vi "英维克通讯.vi"() -> ()   [LabVIEW 2016, in "环境动力监测库.lvlib" / "空调库.lvlib"]
uses:
  <vilib>/Plasmionique/MB Master/MB_Master/MB_Master.lvclass
  <vilib>/Plasmionique/MB Master/MB Master.lvlib
  <vilib>/Utility/config.llb/NI_LVConfig.lvlib
panel:
  out "遥控开关机状态":bool
  out "系统参数":T1
  out "告警状态":T2
  out "传感器状态":T3
  out "运行状态":T4
  out "遥控参数":u16[](array[numeric])
  out "系统参数":u16[](array[numeric])
  out "告警状态":u16[](array[numeric])
  out "传感器状态":u16[](array[numeric])
  out "运行状态":u16[](array[numeric])
  in  "读取参数":bool
  in  "读取数据":bool
  in  "释放串口":bool
  in  "打开串口":bool
  out "队列中元素数量":i32
  out "元素":cluster{"命令":string}[](array[cluster])
  out "待处理插入数量":i32
  out "读取公式":u16[](array[numeric])
  out "读取参数":u16[](array[numeric])
  out "数据存储":u16[](array[numeric])
  out "通讯状态":bool
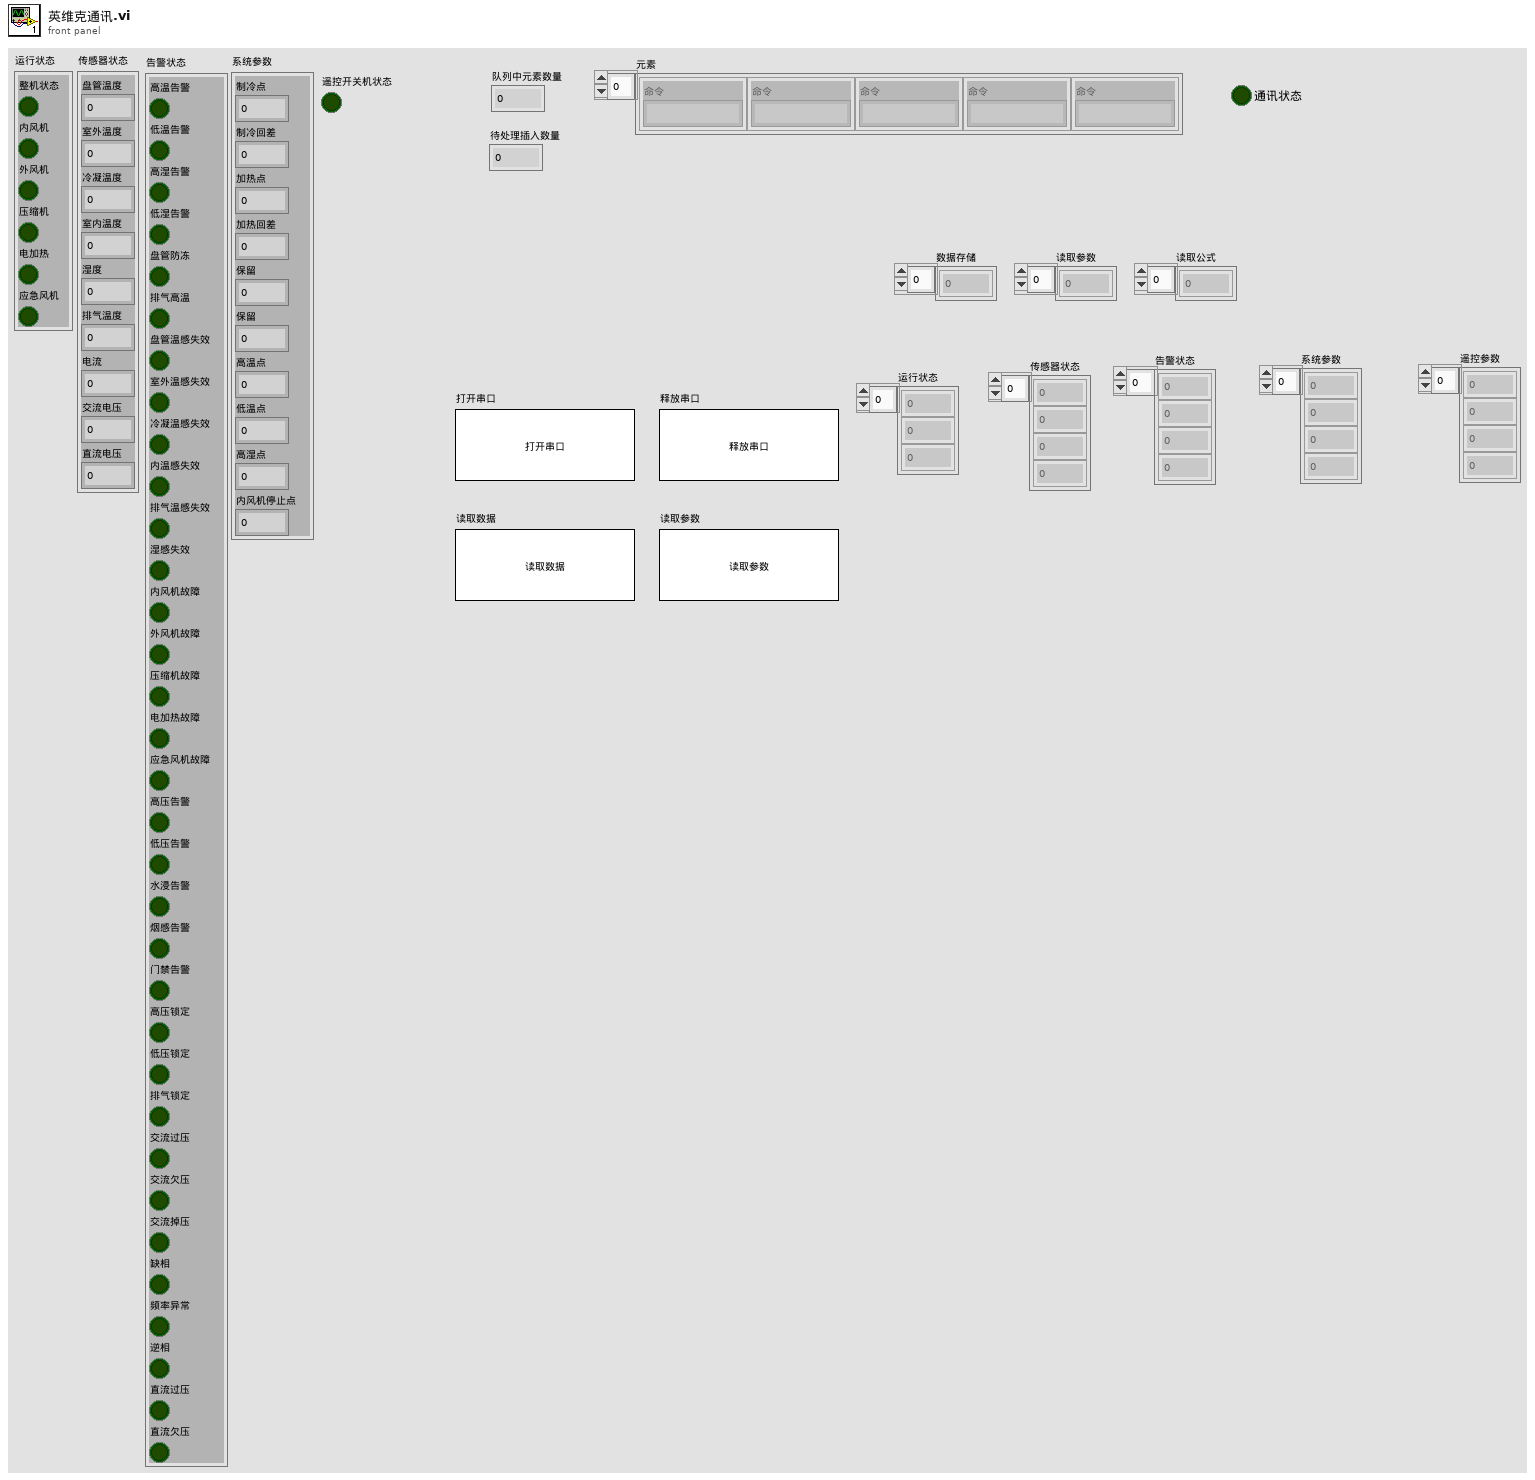
[diagram p1: front panel]
types:
  T1 = cluster{"制冷点":u16, "制冷回差":u16, "加热点":u16, "加热回差":u16, "保留":u16, "保留":u16, "高温点":u16, "低温点":u16, "高湿点":u16, "内风机停止点":u16}
  T2 = cluster{"高温告警":bool, "低温告警":bool, "高湿告警":bool, "低湿告警":bool, "盘管防冻":bool, "排气高温":bool, "盘管温感失效":bool, "室外温感失效":bool, "冷凝温感失效":bool, "内温感失效":bool, "排气温感失效":bool, "湿感失效":bool, "内风机故障":bool, "外风机故障":bool, "压缩机故障":bool, "电加热故障":bool, "应急风机故障":bool, "高压告警":bool, "低压告警":bool, "水浸告警":bool, "烟感告警":bool, "门禁告警":bool, "高压锁定":bool, "低压锁定":bool, "排气锁定":bool, "交流过压":bool, "交流欠压":bool, "交流掉压":bool, "缺相":bool, "频率异常":bool, "逆相":bool, "直流过压":bool, "直流欠压":bool}
  T3 = cluster{"盘管温度":u16, "室外温度":u16, "冷凝温度":u16, "室内温度":u16, "湿度":u16, "排气温度":u16, "电流":u16, "交流电压":u16, "直流电压":u16}
  T4 = cluster{"整机状态":bool, "内风机":bool, "外风机":bool, "压缩机":bool, "电加热":bool, "应急风机":bool}
  T5 = typedef "NI_LVConfig.lvlib/Config Data RefNum.ctl" = refnum<k1>
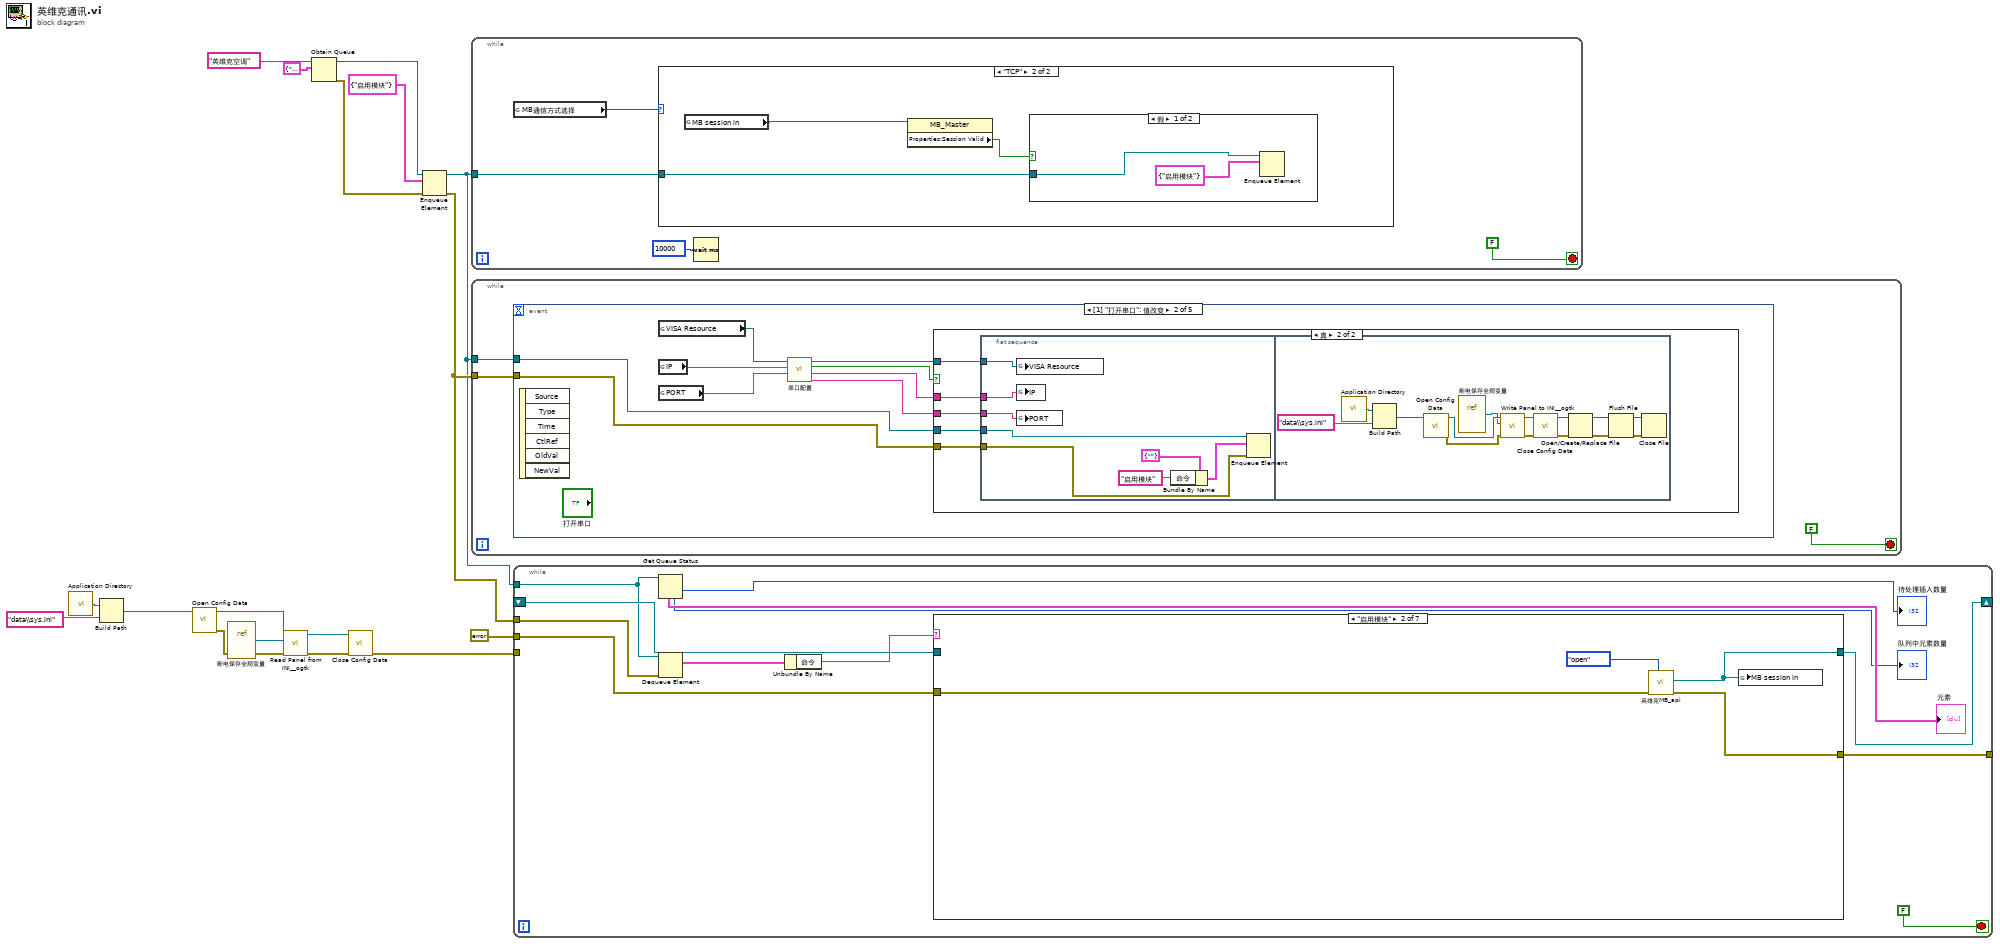
[diagram p0: block diagram]
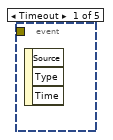
[diagram p4: hidden frame]
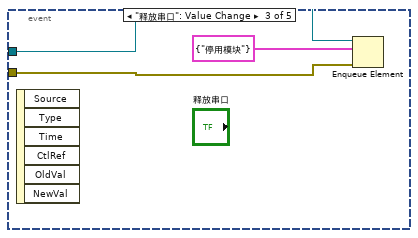
[diagram p6: hidden frame]
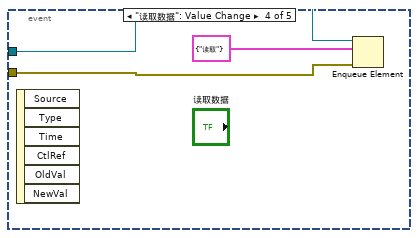
[diagram p7: hidden frame]
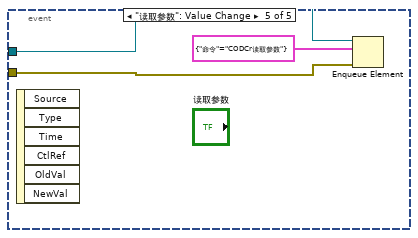
[diagram p8: hidden frame]
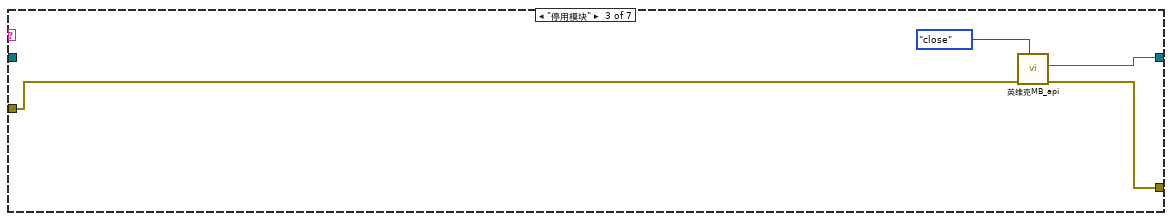
[diagram p10: hidden frame]
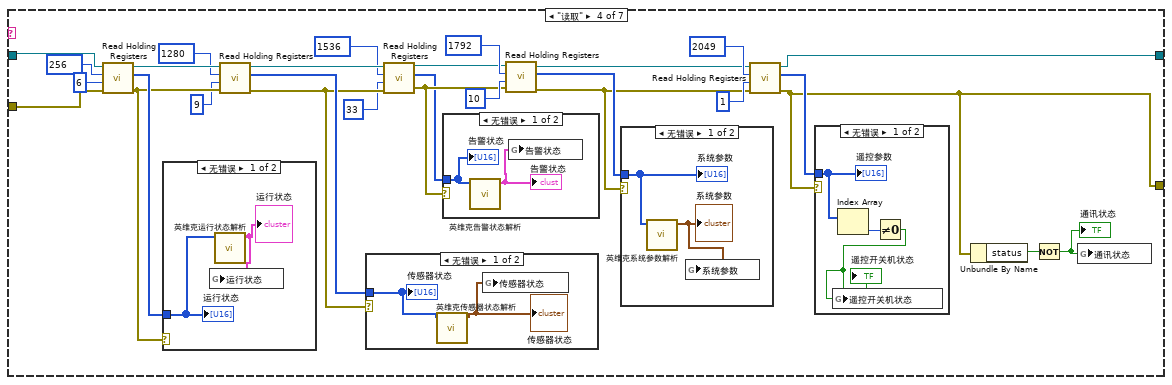
[diagram p11: hidden frame]
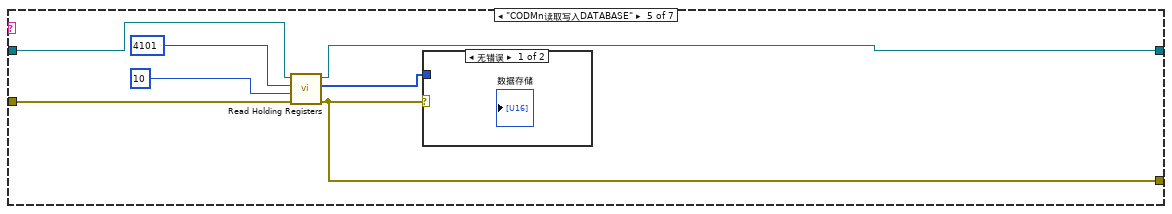
[diagram p17: hidden frame]
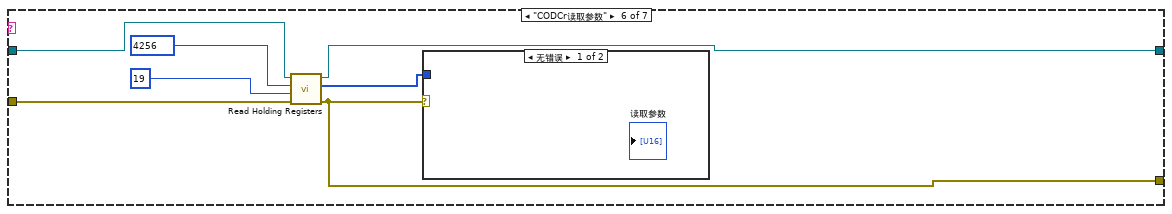
[diagram p19: hidden frame]
diagram:
  n1 = call <vilib>:"Application Directory.vi"() -> ("Application Directory"=w2:path)
  n2 = Build Path(base path=w2, name or relative path="data\\sys.ini" ("名称或相对路径")) -> (appended path=w3:path)
  n3 = call <vilib>:"Open Config Data.vi"("configuration file path"=w3) -> ("error out"=w8:errorcluster, "refnum"=w11:T5)  [unwired: 8 in, 1 out]
  n4 = vi-ref "断电保存全局变量.vi"() -> (w10:refnum<vi>)
  n5 = call <userlib>:"Read Panel from INI__ogtk.vi"("error in (no error)"=w8, "VI ref"=w10, "refnum"=w11) -> ("error out"=w7:errorcluster, "refnum out"=w9:T5)  [unwired: 7 in]
  n6 = Obtain Queue(name (unnamed)="英维克空调" ("名称（未命名）"), element data type=cluster{"命令":string} {"命令"="启用模块"} ("元素")) -> (queue out=w14:refnum<queue>, error out=w13:errorcluster)  [unwired: 3 in, 1 out]
  n7 = call <vilib>:"Close Config Data.vi"("error in (no error)"=w7, "refnum"=w9) -> ("error out"=w4:errorcluster)  [unwired: 8 in, 1 out]
  n8 = Enqueue Element(queue=w14, element=cluster{"命令":string} {"命令"="启用模块"} ("元素"), error in (no error)=w13) -> (queue out=w5:refnum<queue>, error out=w6:errorcluster)  [unwired: 1 in, 1 out]
  n9 = while {
    tunnel: w5 -> [w21]
    stop <- FALSE stop-if-true
    n10 = global read "断电保存全局变量.vi" "MB通信方式选择"() -> (w19:enum16{"串口", "TCP"})
    n11 = case shown="\"TCP\"" w19 {
      tunnel: w21 -> [_ w23]
      frame "串口", Default {
      }
      frame "TCP" {
        n12 = global read "断电保存全局变量.vi" "MB session in"() -> (w22:refnum<class "MB_Master.lvclass">)
        n13 = property class="MB_Master"(reference=w22) -> ("Properties:Session Valid"=w24:bool)  [unwired: 1 in, 2 out]
        n14 = case shown="假" w24 {
          tunnel: w23 -> [w26 _]
          frame False {
            n15 = Enqueue Element(queue=w26, element=cluster{"命令":string} {"命令"="启用模块"} ("元素")) -> ()  [unwired: 2 in, 3 out]
          }
          frame True {
          }
        }
      }
    }
    n16 = Wait (ms)(milliseconds to wait=u32 10000 ("等待时间（毫秒）")) -> ()  [unwired: 1 out]
  }
  n17 = while {
    tunnel: w5 -> [w28]
    tunnel: w6 -> [w27]
    stop <- FALSE stop-if-true
    n18 = event shown="[1] \"打开串口\": 值改变" {
      selector: _ -> [_ _ _ _ _]
      dyn-events: _ -> [_ _ _ _ _]
      timeout: _ -> [_ _ _ _ _]
      tunnel: w28 -> [_ w38 w68 w70 w73]
      tunnel: w27 -> [_ w37 w67 w69 w72]
      event Timeout {
        n19 = event-data() -> ()  [unwired: 1 in, 3 out]
      }
      event "打开串口": Value Change {
        n20 = event-data() -> ()  [unwired: 1 in, 6 out]
        n21 = global read "断电保存全局变量.vi" "VISA Resource"() -> (w36:refnum<visa-resource-name>)
        n22 = global read "断电保存全局变量.vi" "IP"() -> (w31:string)
        n23 = global read "断电保存全局变量.vi" "PORT"() -> (w30:string)
        n24 = call "串口配置.vi"("PORT"=w30, "IP"=w31, "请选择串口:"=w36) -> ("PORT 2"=w32:string, "IP 2"=w33:string, "确认 2"=w34:bool, "VISA资源名称 2"=w35:refnum<visa-resource-name>)  [unwired: 5 in]
        n25 = case shown="真" w34 {
          tunnel: w35 -> [_ w41]
          tunnel: w38 -> [_ w43]
          tunnel: w37 -> [_ w42]
          tunnel: w33 -> [_ w40]
          tunnel: w32 -> [_ w39]
          frame False {
          }
          frame True {
            n26 = flat-sequence {
              tunnel: w43 -> [w48]
              tunnel: w42 -> [w47]
              tunnel: w41 -> [w46]
              tunnel: w40 -> [w45]
              tunnel: w39 -> [w44]
              frame #0 {
                n27 = global write "断电保存全局变量.vi" "VISA Resource"(w46) -> ()
                n28 = global write "断电保存全局变量.vi" "IP"(w45) -> ()
                n29 = global write "断电保存全局变量.vi" "PORT"(w44) -> ()
                n30 = Bundle By Name(cluster=cluster{"命令":string} {"命令"=""} ("元素"), "命令"="启用模块" ("名称（未命名）")) -> (w49:cluster{"命令":string})
                n31 = Enqueue Element(queue=w48, element=w49, error in (no error)=w47) -> ()  [unwired: 1 in, 3 out]
              }
              frame #1 {
                n32 = call <vilib>:"Application Directory.vi"() -> ("Application Directory"=w64:path)
                n33 = Build Path(base path=w64, name or relative path="data\\sys.ini" ("名称或相对路径")) -> (appended path=w63:path)
                n34 = call <vilib>:"Open Config Data.vi"("configuration file path"=w63) -> ("error out"=w59:errorcluster, "refnum"=w62:T5)  [unwired: 8 in, 1 out]
                n35 = vi-ref "断电保存全局变量.vi"() -> (w61:refnum<vi>)
                n36 = call <userlib>:"Write Panel to INI__ogtk.vi"("error in (no error)"=w59, "VI ref"=w61, "refnum"=w62) -> ("error out"=w58:errorcluster, "refnum out"=w60:T5)  [unwired: 7 in]
                n37 = call <vilib>:"Close Config Data.vi"("error in (no error)"=w58, "refnum"=w60) -> ("error out"=w53:errorcluster, "file path"=w52:path)  [unwired: 8 in]
                n38 = Open/Create/Replace File(file path (use dialog)=w52, error in=w53) -> (refnum out=w56:refnum<file>, error out=w57:errorcluster)  [unwired: 4 in, 1 out]
                n39 = Flush File(refnum=w56, error in=w57) -> (refnum out=w55:refnum<file>, error out=w54:errorcluster)
                n40 = Close File(refnum=w55, error in=w54) -> ()  [unwired: 2 out]
              }
            }
          }
        }
      }
      event "释放串口": Value Change {
        n41 = event-data() -> ()  [unwired: 1 in, 6 out]
        n42 = Enqueue Element(queue=w68, element=cluster{"命令":string} {"命令"="停用模块"} ("元素"), error in (no error)=w67) -> ()  [unwired: 1 in, 3 out]
      }
      event "读取数据": Value Change {
        n43 = event-data() -> ()  [unwired: 1 in, 6 out]
        n44 = Enqueue Element(queue=w70, element=cluster{"命令":string} {"命令"="读取"} ("元素"), error in (no error)=w69) -> ()  [unwired: 1 in, 3 out]
      }
      event "读取参数": Value Change {
        n45 = event-data() -> ()  [unwired: 1 in, 6 out]
        n46 = Enqueue Element(queue=w73, element=cluster{"命令":string} {"命令"="CODCr读取参数"} ("元素"), error in (no error)=w72) -> ()  [unwired: 1 in, 3 out]
      }
    }
  }
  n47 = while {
    tunnel: w5 -> [w78]
    tunnel: w6 -> [w85]
    tunnel: [w79] -> _
    shift-right: [w82] -> _
    shift-left: _ -> [w81]
    tunnel: errorcluster {"status"=FALSE, "code"=0, "source"=""} ("error out") -> [w80]
    tunnel: w4 -> [_]
    stop <- FALSE stop-if-true
    n48 = Get Queue Status(queue=w78) -> (# pending insert=→"待处理插入数量":i32, # elements in queue=→"队列中元素数量":i32, elements=→"元素":cluster{"命令":string}[])  [unwired: 2 in, 5 out]
    n49 = Dequeue Element(queue=w78, error in (no error)=w85) -> (element=w84:cluster{"命令":string})  [unwired: 1 in, 3 out]
    n50 = Unbundle By Name(w84) -> ("命令"=w83:string)
    n51 = case shown="\"启用模块\"" w83 {
      tunnel: [w88 w89 w93 w98 w139 w147 w154] -> w82
      tunnel: [w87 w92 w94 w97 w137 w146 w153] -> w79
      tunnel: w81 -> [w88 _ _ w125 w143 w150 w157]
      tunnel: w80 -> [w87 w90 w95 w124 w140 w149 w156]
      frame Default {
      }
      frame "启用模块" {
        n52 = call "英维克MB_api.vi"("STEP"=enum16{"open", "read", "write", "close"}."open", "Error in"=w90) -> ("error out"=w92:errorcluster, "MB session out"=w89:refnum<class "MB_Master.lvclass">)  [unwired: 7 in, 1 out]
        n53 = global write "断电保存全局变量.vi" "MB session in"(w89) -> ()
      }
      frame "停用模块" {
        n54 = call "英维克MB_api.vi"("STEP"=enum16{"open", "read", "write", "close"}."close", "Error in"=w95) -> ("error out"=w94:errorcluster, "MB session out"=w93:refnum<class "MB_Master.lvclass">)  [unwired: 7 in, 1 out]
      }
      frame "读取" {
        n55 = call <vilib>:"Read Holding Registers.vi"("error in (no error)"=w124, "quantity"=u16 6 ("number of holding registers"), "starting address"=u16 256, "MB session in"=w125) -> ("error out"=w121:errorcluster, "Registers"=w123:u16[], "MB session out"=w122:refnum<class "MB_Master.lvclass">)  [unwired: 5 in]
        n56 = case shown="无错误" w121 {
          tunnel: w123 -> [w136 _]
          frame No Error {
            n57 = call "英维克运行状态解析.vi"("运行状态输入"=w136) -> ("运行状态"=w135:T4)  [unwired: 10 in]
            "运行状态" <- w135
            n58 = global write "内部交互全局变量.vi" "运行状态"(w135) -> ()
            "运行状态" <- w136
          }
          frame Error {
          }
        }
        n59 = call <vilib>:"Read Holding Registers.vi"("error in (no error)"=w121, "quantity"=u16 9 ("number of holding registers"), "starting address"=u16 1280, "MB session in"=w122) -> ("error out"=w112:errorcluster, "Registers"=w120:u16[], "MB session out"=w113:refnum<class "MB_Master.lvclass">)  [unwired: 5 in]
        n60 = case shown="无错误" w112 {
          tunnel: w120 -> [w134 _]
          frame No Error {
            n61 = call "英维克传感器状态解析.vi"("传感器状态输入"=w134) -> ("传感器状态输出"=w133:T3)  [unwired: 10 in]
            "传感器状态" <- w133
            n62 = global write "内部交互全局变量.vi" "传感器状态"(w133) -> ()
            "传感器状态" <- w134
          }
          frame Error {
          }
        }
        n63 = call <vilib>:"Read Holding Registers.vi"("error in (no error)"=w112, "quantity"=u16 33 ("number of holding registers"), "starting address"=u16 1536, "MB session in"=w113) -> ("error out"=w106:errorcluster, "Registers"=w105:u16[], "MB session out"=w107:refnum<class "MB_Master.lvclass">)  [unwired: 5 in]
        n64 = case shown="无错误" w106 {
          tunnel: w105 -> [w132 _]
          frame No Error {
            n65 = call "英维克告警状态解析.vi"("告警状态输入"=w132) -> ("告警状态"=w131:T2)  [unwired: 10 in]
            "告警状态" <- w131
            n66 = global write "内部交互全局变量.vi" "告警状态"(w131) -> ()
            "告警状态" <- w132
          }
          frame Error {
          }
        }
        n67 = call <vilib>:"Read Holding Registers.vi"("error in (no error)"=w106, "quantity"=u16 10 ("number of holding registers"), "starting address"=u16 1792, "MB session in"=w107) -> ("error out"=w101:errorcluster, "Registers"=w104:u16[], "MB session out"=w100:refnum<class "MB_Master.lvclass">)  [unwired: 5 in]
        n68 = case shown="无错误" w101 {
          tunnel: w104 -> [w130 _]
          frame No Error {
            n69 = call "英维克系统参数解析.vi"("系统参数输入"=w130) -> ("系统参数"=w129:T1)  [unwired: 10 in]
            "系统参数" <- w129
            n70 = global write "内部交互全局变量.vi" "系统参数"(w129) -> ()
            "系统参数" <- w130
          }
          frame Error {
          }
        }
        n71 = call <vilib>:"Read Holding Registers.vi"("error in (no error)"=w101, "quantity"=u16 1 ("number of holding registers"), "starting address"=u16 2049, "MB session in"=w100) -> ("error out"=w97:errorcluster, "Registers"=w99:u16[], "MB session out"=w98:refnum<class "MB_Master.lvclass">)  [unwired: 5 in]
        n72 = case shown="无错误" w97 {
          tunnel: w99 -> [w128 _]
          frame No Error {
            n73 = Index Array(array=w128) -> (element=w127:u16)  [unwired: 1 in]
            n74 = Not Equal To 0?(x=w127) -> (x != 0?=w126:bool)
            "遥控开关机状态" <- w126
            n75 = global write "内部交互全局变量.vi" "遥控开关机状态"(w126) -> ()
            "遥控参数" <- w128
          }
          frame Error {
          }
        }
        n76 = Unbundle By Name(w97) -> ("status"=w114:bool)
        n77 = Not(x=w114) -> (.not. x?=w115:bool)
        "通讯状态" <- w115
        n78 = global write "断电保存全局变量.vi" "通讯状态"(w115) -> ()
      }
      frame "CODMn读取写入DATABASE" {
        n79 = call <vilib>:"Read Holding Registers.vi"("error in (no error)"=w140, "quantity"=u16 10 ("number of holding registers"), "starting address"=u16 4101, "MB session in"=w143) -> ("error out"=w137:errorcluster, "Registers"=w138:u16[], "MB session out"=w139:refnum<class "MB_Master.lvclass">)  [unwired: 5 in]
        n80 = case shown="无错误" w137 {
          tunnel: w138 -> [_ _]
          frame No Error {
          }
          frame Error {
          }
        }
      }
      frame "CODCr读取参数" {
        n81 = call <vilib>:"Read Holding Registers.vi"("error in (no error)"=w149, "quantity"=u16 19 ("number of holding registers"), "starting address"=u16 4256, "MB session in"=w150) -> ("error out"=w146:errorcluster, "Registers"=w148:u16[], "MB session out"=w147:refnum<class "MB_Master.lvclass">)  [unwired: 5 in]
        n82 = case shown="无错误" w146 {
          tunnel: w148 -> [_ _]
          frame No Error {
          }
          frame Error {
          }
        }
      }
      frame "CODMn读取公式" {
        n83 = call <vilib>:"Read Holding Registers.vi"("error in (no error)"=w156, "quantity"=u16 94 ("number of holding registers"), "starting address"=u16 4616, "MB session in"=w157) -> ("error out"=w153:errorcluster, "Registers"=w155:u16[], "MB session out"=w154:refnum<class "MB_Master.lvclass">)  [unwired: 5 in]
        n84 = case shown="无错误" w153 {
          tunnel: w155 -> [_ _]
          frame No Error {
          }
          frame Error {
          }
        }
      }
    }
  }
